vi "DriveAtAngle.vi"(0 "Target Angle":dbl, 1 "Distance":dbl, 3 "Error In":errorcluster) -> (7 "y-axis distance":dbl, 8 "x":dbl, 9 "y":dbl, 10 "Error Out":errorcluster)   [LabVIEW 2017]
panel:
  out "x power":dbl
  out "y power":dbl
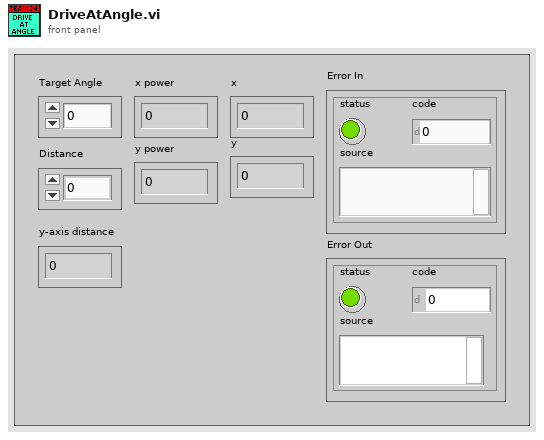
[diagram p1: front panel]
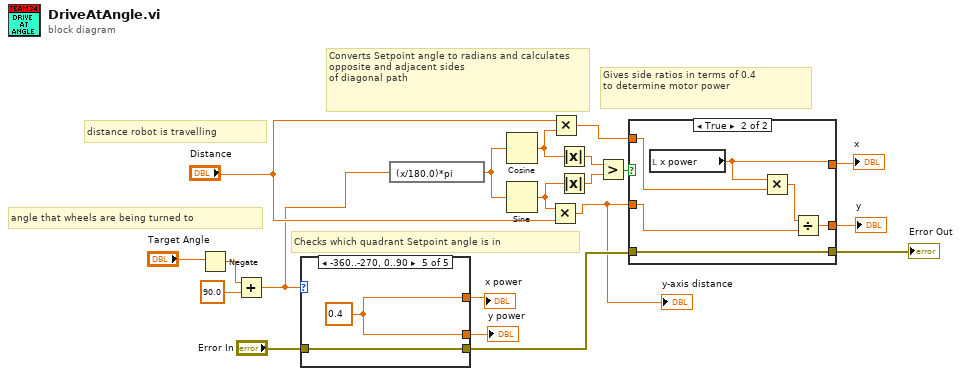
[diagram p0: block diagram]
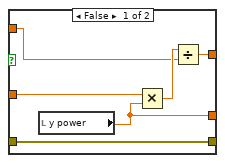
[diagram p2: hidden frame]
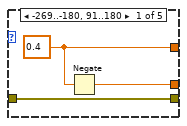
[diagram p3: hidden frame]
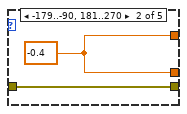
[diagram p4: hidden frame]
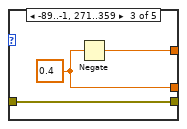
[diagram p5: hidden frame]
diagram:
  # "Checks which quadrant Setpoint angle is in"
  # "Gives side ratios in terms of 0.4\nto determine motor power"
  # "Converts Setpoint angle to radians and calculates opposite and adjacent sides \nof diagonal path"
  # "distance robot is travelling"
  # "angle that wheels are being turned to"
  n1 = Negate(x="Target Angle") -> (-x=w15:dbl)
  n2 = Add(x=w15, y=90.0) -> (x+y=w14:dbl)
  n3 = case shown="-360..-270, 0..90" w14 {
    tunnel: [w23 w25 w28 _ w31] -> w17
    tunnel: [w22 w25 w27 _ w31] -> w18
    tunnel: "Error In" -> [w21 w24 w26 w29 w30]
    tunnel: [w21 w24 w26 w29 w30] -> w6
    frame -269..-180, 91..180 {
      w22 = 0.4 ("x power")
      n4 = Negate(x=w22) -> (-x=w23:dbl)
    }
    frame -179..-90, 181..270 {
      w25 = -0.4 ("x power")
    }
    frame -89..-1, 271..359 {
      w28 = 0.4 ("x power")
      n5 = Negate(x=w28) -> (-x=w27:dbl)
    }
    frame Default {
    }
    frame -360..-270, 0..90 {
      w31 = 0.4 ("x power")
    }
  }
  "x power" <- w18
  "y power" <- w17
  n6 = expression code="(x/180.0)*pi"(w14) -> (w20:dbl)
  n7 = Cosine(x=w20) -> (cos(x)=w11:dbl)
  n8 = Sine(x=w20) -> (sin(x)=w10:dbl)
  n9 = Multiply(x=w10, y="Distance") -> (x*y=w1:dbl)
  "y-axis distance" <- w1
  n10 = Multiply(x="Distance", y=w11) -> (x*y=w12:dbl)
  n11 = Absolute Value(x=w11) -> (abs(x)=w8:dbl)
  n12 = Absolute Value(x=w10) -> (abs(x)=w9:dbl)
  n13 = Greater?(x=w8, y=w9) -> (0:w5:bool)
  n14 = case shown="True" w5 {
    tunnel: [w37 w42] -> w4
    tunnel: [w36 w41] -> w3
    tunnel: w1 -> [w34 w40]
    tunnel: w12 -> [w33 w39]
    tunnel: w6 -> [w32 w38]
    tunnel: [w32 w38] -> w2
    frame False {
      n15 = local read "y power"() -> (w37:dbl)
      n16 = Multiply(x=w34, y=w37) -> (x*y=w35:dbl)
      n17 = Divide(x=w35, y=w33) -> (x/y=w36:dbl)
    }
    frame True {
      n18 = local read "x power"() -> (w41:dbl)
      n19 = Multiply(x=w41, y=w39) -> (x*y=w43:dbl)
      n20 = Divide(x=w43, y=w40) -> (x/y=w42:dbl)
    }
  }
  "Error Out" <- w2
  "x" <- w3
  "y" <- w4
